vi "FromRepo.vi"(8 "error in":errorcluster, 9 "from repo cluster":T2, 10 "repository in":refnum<class "NISE_CEF_Repository.lvclass">, 11 "node in":refnum<class "Targets.lvclass">) -> (0 "error out":errorcluster, 2 "repository out":refnum<class "NISE_CEF_Repository.lvclass">, 3 "node":T1)   [LabVIEW 2013, in "PL Framework Configuration Tool.lvlib" / "Targets.lvclass"]
doc: "Grabs information from the Repo and stores it in the nodes."
uses:
  Targets.lvclass
  <vilib>/NI/Configuration Framework/Repository/NISE_CEF_Repository.lvclass
  <vilib>/NI/Configuration Framework/Node/FromRepoCluster.ctl
  <vilib>/NI/Configuration Framework/Node/NodeRef.ctl
  <vilib>/NI/Configuration Framework/Node/NISE_CEF_Node.lvclass
  TBM Configuration Node/deployment configuration.ctl
  TBM Configuration Node/TBM Configuration Node.lvclass
  Framework Configuration Classes/target configuration/PL_Target Configuration.lvclass/PL_Target Configuration.ctl
  Targets.lvclass/Targets.ctl
  Write local bitfile path.vi
  Write additional files.vi
  read target configuration.vi
  Framework Configuration Classes/target configuration/PL_Target Configuration.lvclass
  <vilib>/NI/Configuration Framework/serializable configuration/NISE_CEF_serializable configuration.lvclass
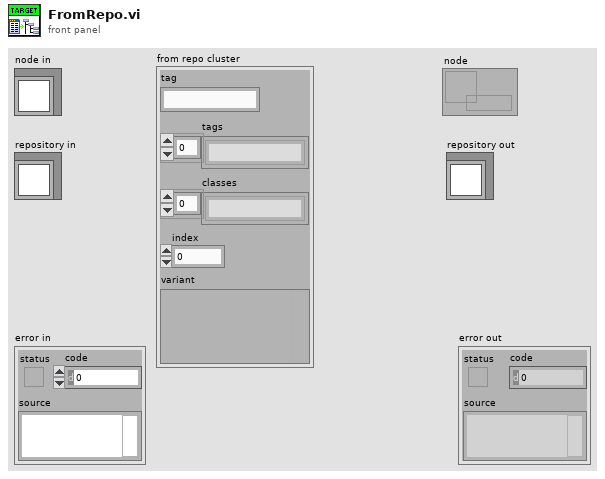
[diagram p1: front panel]
types:
  T1 = typedef "NISE_CEF_Node.lvclass/NodeRef.ctl" = refnum<data-value>
  T2 = typedef "NISE_CEF_Node.lvclass/FromRepoCluster.ctl" = cluster{"tag":string, "tags":string[], "classes":string[], "index":i32, "variant":variant}
  T3 = typedef "PL Framework Configuration Tool.lvlib/TBM Configuration Node.lvclass/deployment configuration.ctl" = cluster{"local path":path, "remote path (relative to root)":path}
  T4 = typedef "TBM configuration.lvclass/Target Types.ctl" = enum16{"Windows", "Mac", "Linux", "Linux RT ARM", "VxWorks", "Pharlap", "Other", "Linux RT x64"}
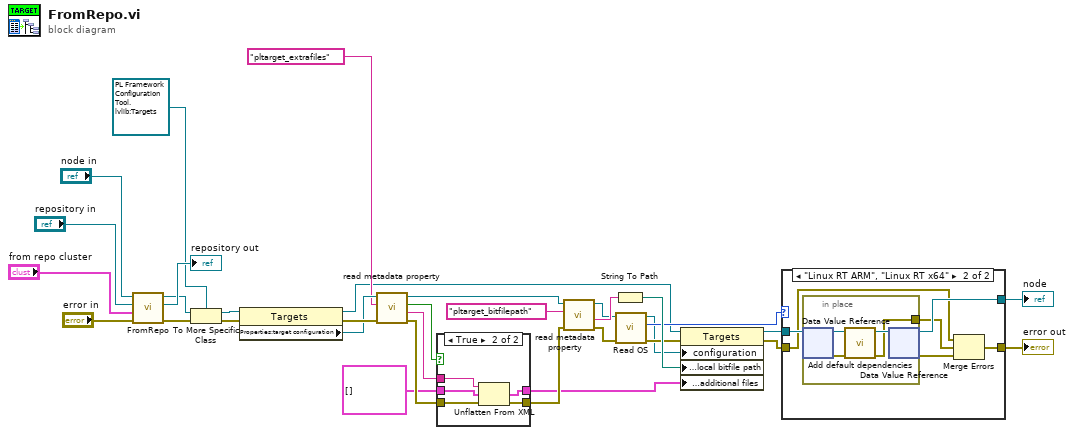
[diagram p0: block diagram]
diagram:
  n1 = call-parent "FromRepo.vi"("error in"="error in", "from repo cluster"="from repo cluster", "repository in"="repository in", "node in"="node in") -> ("error out"=w32:errorcluster, "repository out"=→"repository out":refnum<class "NISE_CEF_Repository.lvclass">, "node"=w30:T1)  [unwired: 5 in]
  n2 = To More Specific Class(target class=refnum<data-value> refnum, reference=w30, error in=w32) -> (specific class reference=w29:refnum<data-value>, error out=w31:errorcluster)
  n3 = property class="Targets"(reference=w29, error in=w31) -> (reference out=w7:refnum<data-value>, error out=w25:errorcluster, "Properties:target configuration"=w18:refnum<class "PL_Target Configuration.lvclass">)
  n4 = call <vilib>:"read metadata property.vi"("error in"=w25, "key"="pltarget_extrafiles", "configuration in"=w18) -> ("error out"=w19:errorcluster, "value"=w12:string, "found"=w13:bool, "configuration out"=w17:refnum<class "PL_Target Configuration.lvclass">)  [unwired: 5 in]
  n5 = case shown="True" w13 {
    tunnel: w19 -> [w35 w40]
    tunnel: [w35 w39] -> w16
    tunnel: T3[] [] ("additional files") -> [w34 w38]
    tunnel: [w34 w37] -> w14
    tunnel: w12 -> [_ w36]
    frame False {
    }
    frame True {
      n6 = Unflatten From XML(xml string=w36, type=w38, error in (no error)=w40) -> (value=w37:T3[], error out=w39:errorcluster)
    }
  }
  n7 = call <vilib>:"read metadata property.vi"("error in"=w16, "key"="pltarget_bitfilepath", "configuration in"=w17) -> ("error out"=w9:errorcluster, "value"=w26:string, "configuration out"=w10:refnum<class "PL_Target Configuration.lvclass">)  [unwired: 5 in, 1 out]
  n8 = String To Path(string=w26) -> (path=w24:path)
  n9 = call "Read OS.vi"("error in"=w9, "PL_Target Configuration in"=w10) -> ("error out"=w6:errorcluster, "Target Types"=w8:T4, "PL_Target Configuration out"=w5:refnum<class "PL_Target Configuration.lvclass">)  [unwired: 7 in]
  n10 = property class="Targets"(reference=w7, error in=w6, "configuration"=w5, "data access:local bitfile path"=w24, "data access:additional files"=w14) -> (reference out=w4:refnum<data-value>, error out=w2:errorcluster)
  n11 = case shown="\"Linux RT ARM\", \"Linux RT x64\"" w8 {
    tunnel: w4 -> [w42 w48]
    tunnel: [w42 w47] -> w3
    tunnel: w2 -> [w41 w46]
    tunnel: [w41 w45] -> w1
    frame Default {
    }
    frame "Linux RT ARM", "Linux RT x64" {
      n12 = in-place {
        in-place-border: [w49] -> w44
        n13 = in-place-dvr #1(w48) -> (w52:refnum<class "Targets.lvclass">, w50:errorcluster)
        n14 = call "Add default dependencies.vi"("error in (no error)"=w50, "Targets in"=w52) -> ("error out"=w49:errorcluster, "Targets out"=w51:refnum<class "Targets.lvclass">)  [unwired: 8 in]
        n15 = in-place-dvr #1(w51) -> (w47:refnum<data-value>, w43:errorcluster)
      }
      n16 = Merge Errors(w46, w44, w43) -> (w45:errorcluster)
    }
  }
  "error out" <- w1
  "node" <- w3
